vi "click_button.vi"(4 "ButtonLabel":string) -> ()   [LabVIEW 2016]
panel:
  out "error out":errorcluster
  in  "error in":errorcluster
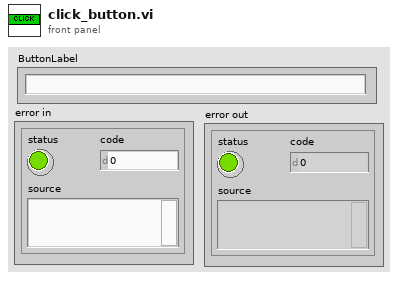
[diagram p1: front panel]
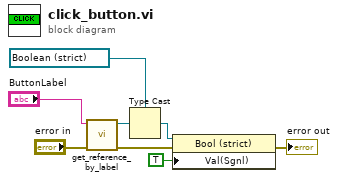
[diagram p0: block diagram]
diagram:
  n1 = call "get_reference_by_label.vi"("error in"="error in", "Label"="ButtonLabel") -> ("error out"=w6:errorcluster, "Ctl Refnum"=w8:refnum<vi>)  [unwired: 7 in, 1 out]
  n2 = Type Cast(type=refnum<vi> refnum ("PA"), x=w8) -> (*(type *) &x=w7:refnum<vi>)
  n3 = property class="Bool (strict)"(reference=w7, error in=w6, "Val(Sgnl)"=TRUE ("Value (Signaling)")) -> (error out=→"error out":errorcluster)  [unwired: 1 out]
